vi "Config Dialog.vi"(10 "Container State":T1 caption="container state", 11 "state in":T2={"Draw Options"={"Outer Border Color"=0, "Inner Border Color"=6316128, "Outer Gradient Color"=2565927, "Inner Gradient Color"=16860, "Compass North Pointer Color"=16711680, "Compass Pointer Color 1"=13355429, "Compass Pointer Color 2"=14934973, "Direction Pointer Color"=16765184, "Text Box Outline Color"=13355429, "Text Box Background Color"=14934973, "Scale Color"=16448250, "Text Color"=0, "Draw Gradient"=TRUE, "Draw Rose"=TRUE, "Simple Scale"=TRUE, "Draw Text"=FALSE, "Font Name"="Helvetica", "Angle Units"=enum."Degrees"}} caption="State") -> (0 "state changed?":bool, 1 "data changed?":bool, 3 "state out":T2={"Draw Options"={"Outer Border Color"=0, "Inner Border Color"=6316128, "Outer Gradient Color"=2565927, "Inner Gradient Color"=16860, "Compass North Pointer Color"=16711680, "Compass Pointer Color 1"=13355429, "Compass Pointer Color 2"=14934973, "Direction Pointer Color"=16765184, "Text Box Outline Color"=13355429, "Text Box Background Color"=14934973, "Scale Color"=16448250, "Text Color"=0, "Draw Gradient"=TRUE, "Draw Rose"=TRUE, "Simple Scale"=TRUE, "Draw Text"=FALSE, "Font Name"="Helvetica", "Angle Units"=enum."Degrees"}} caption="State")   [LabVIEW 2017, in "Compass Indicator.xctl"]
uses:
  <vilib>/robotics/Controls/Compass Indicator/Compass Indicator.xctl
  <vilib>/robotics/Controls/Utilities/Color Box.ctl
  <vilib>/robotics/Controls/Compass Indicator/_Compass Indicator Support Files/Compass State.ctl
  <vilib>/robotics/Controls/Compass Indicator/Compass Picture/Draw Options.ctl
  <vilib>/robotics/Controls/Utilities/Angle Units.ctl
  <vilib>/_xctls/Container State.ctl
  <vilib>/robotics/Controls/Compass Indicator/Compass Picture/NI_Robotics_Compass Picture.lvlib
  <vilib>/_xctls/XControlSupport.lvlib
  <vilib>/robotics/Controls/Utilities/NI_Robotics_Control Utilities.lvlib
panel:
  in  "help":bool
  in  "cancel":bool
  in  "ok":bool
  in  "Angle Units":enum16{"Radians", "Degrees"}(ring)=enum."Degrees"
  out "2D Picture":picture
  in  "draw text":bool caption="Draw Text"
  in  "draw simple scale":bool=TRUE caption="Draw Simple Scale"
  in  "draw rose":bool=TRUE caption="Draw Rose"
  in  "draw grad":bool=TRUE caption="Draw Gradient"
  in  "text color":T5 caption="Text"
  in  "scale color":T5=16448250 caption="Scale"
  in  "text box bkgnd color":T5=14934973 caption="Text Box Background"
  in  "text box outline color":T5=13355429 caption="Text Box Outline"
  in  "dir ptr color":T5=16765184 caption="Direction Pointer"
  in  "compass ptr 2 color":T5=14934973 caption="Compass Pointer 2"
  in  "compass ptr1 color":T5=13355429 caption="Compass Pointer 1"
  in  "compass north ptr color":T5=16711680 caption="Compass North Pointer"
  in  "inner grad color":T5=16860 caption="Inner Gradient"
  in  "outer grad color":T5=2565927 caption="Outer Gradient"
  in  "inner border color":T5=6316128 caption="Inner Border"
  in  "outer border color":T5 caption="Outer Border"
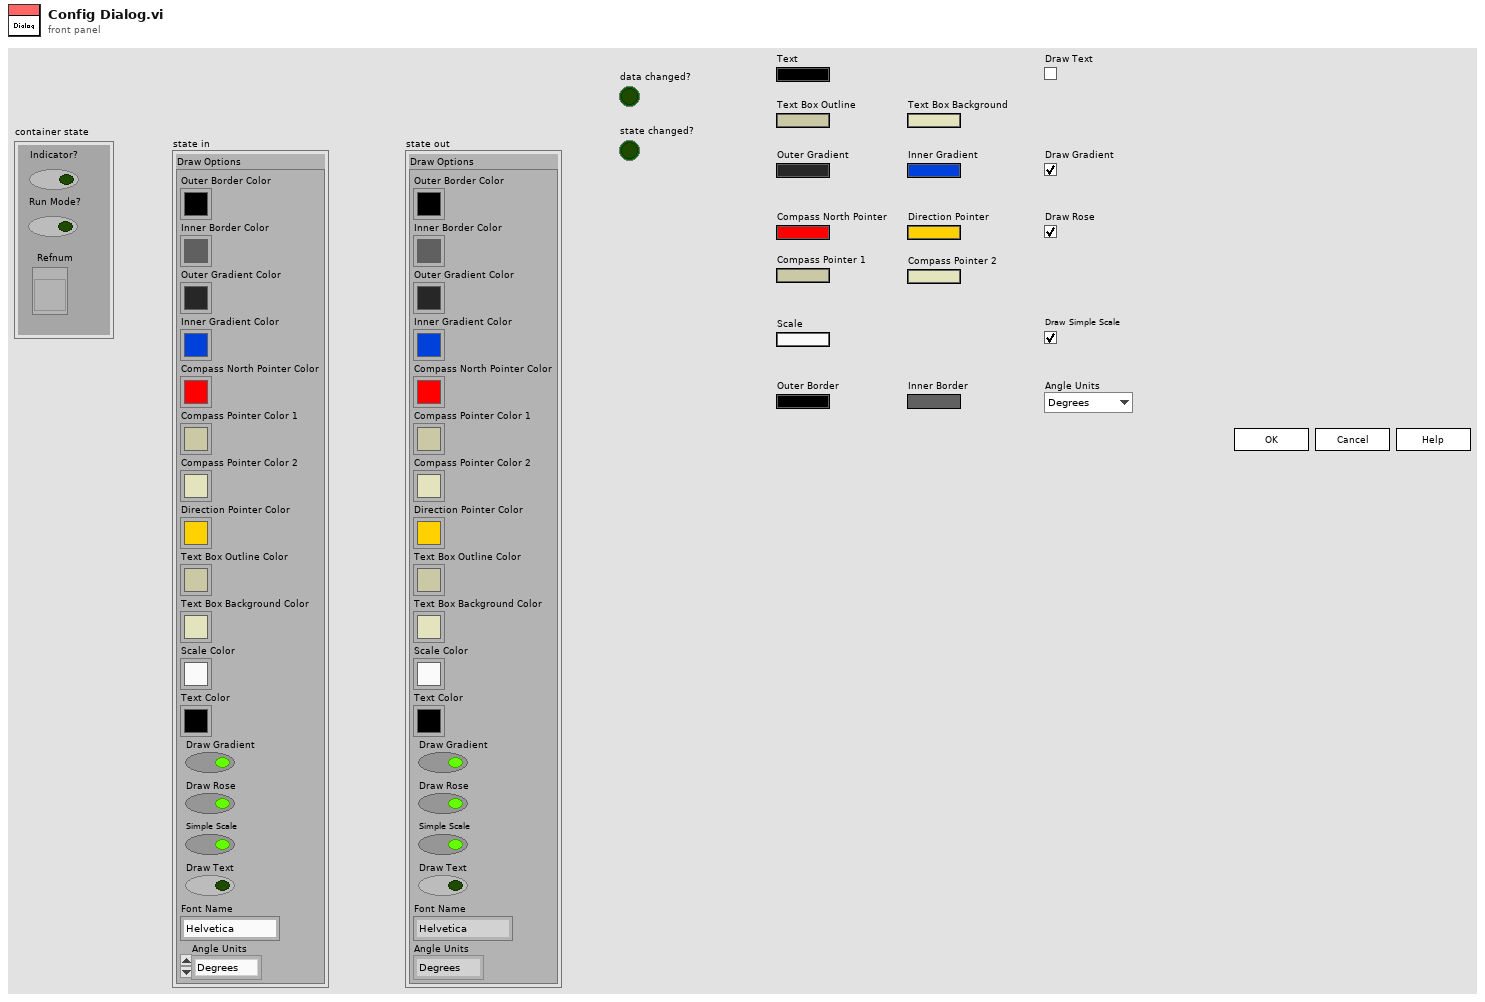
[diagram p1: front panel]
types:
  T1 = typedef "XControlSupport.lvlib/Container State.ctl" = cluster{"Indicator?":bool, "Run Mode?":bool, " Refnum":refnum<vi>}
  T2 = typedef "Compass Indicator.xctl/Compass State.ctl" = cluster{"Draw Options":T3}
  T3 = typedef "NI_Robotics_Compass Picture.lvlib/Draw Options.ctl" = cluster{"Outer Border Color":u32, "Inner Border Color":u32, "Outer Gradient Color":u32, "Inner Gradient Color":u32, "Compass North Pointer Color":u32, "Compass Pointer Color 1":u32, "Compass Pointer Color 2":u32, "Direction Pointer Color":u32, "Text Box Outline Color":u32, "Text Box Background Color":u32, "Scale Color":u32, "Text Color":u32, "Draw Gradient":bool, "Draw Rose":bool, "Simple Scale":bool, "Draw Text":bool, "Font Name":string, "Angle Units":T4}
  T4 = typedef "NI_Robotics_Control Utilities.lvlib/Angle Units.ctl" = enum16{"Radians", "Degrees"}
  T5 = typedef "NI_Robotics_Control Utilities.lvlib/Color Box.ctl" = u32
  T6 = typedef "LVBoundsTypeDef.ctl" = cluster{"Width":u32, "Height":u32}
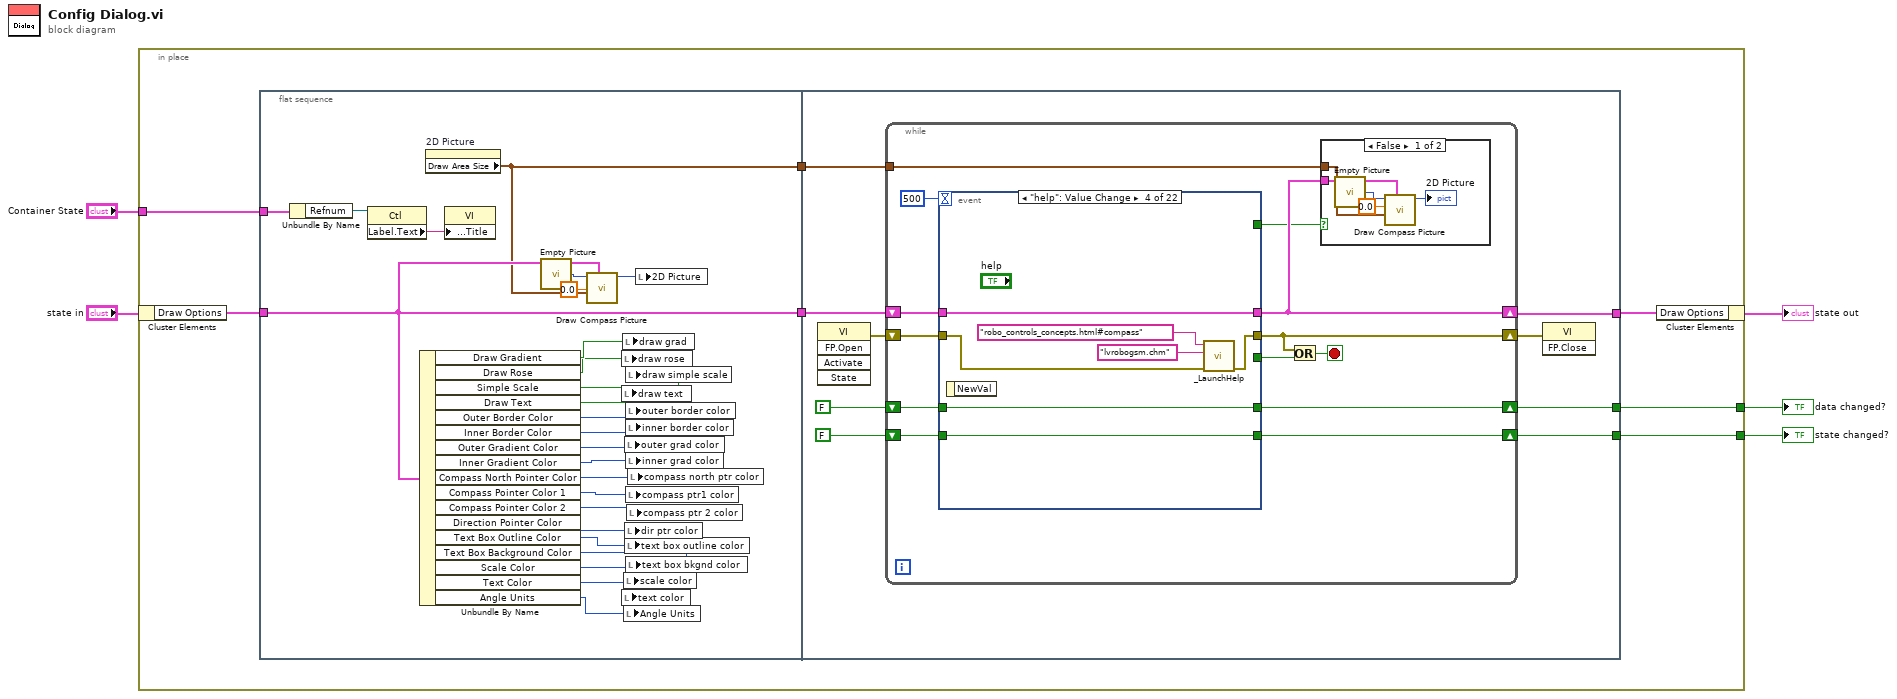
[diagram p0: block diagram]
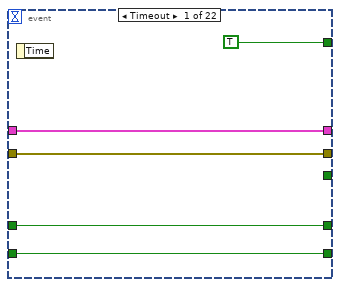
[diagram p3: hidden frame]
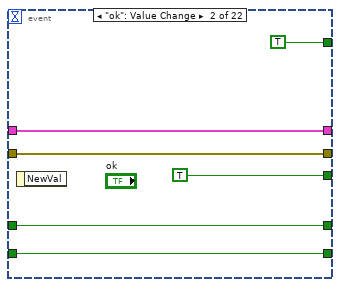
[diagram p4: hidden frame]
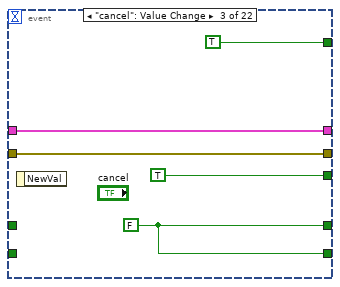
[diagram p5: hidden frame]
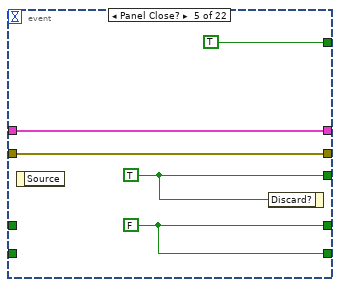
[diagram p6: hidden frame]
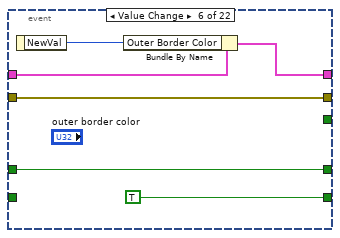
[diagram p7: hidden frame]
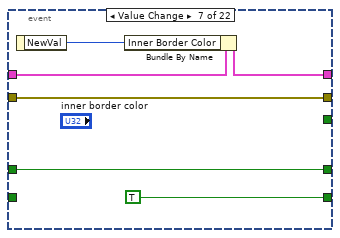
[diagram p8: hidden frame]
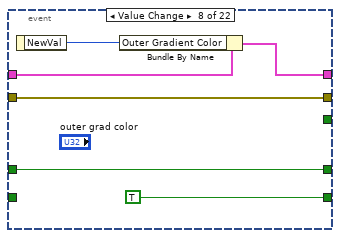
[diagram p9: hidden frame]
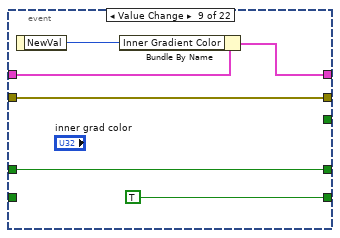
[diagram p10: hidden frame]
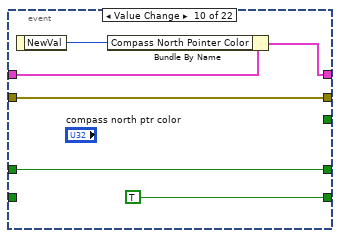
[diagram p11: hidden frame]
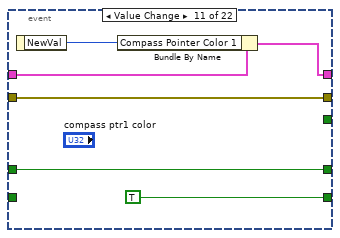
[diagram p12: hidden frame]
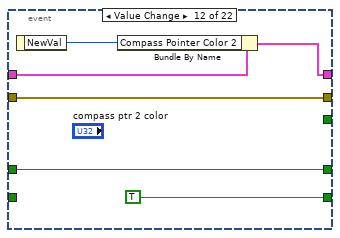
[diagram p13: hidden frame]
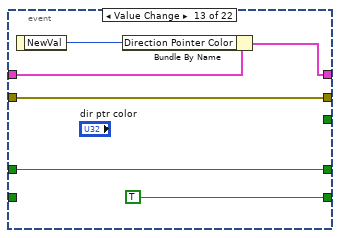
[diagram p14: hidden frame]
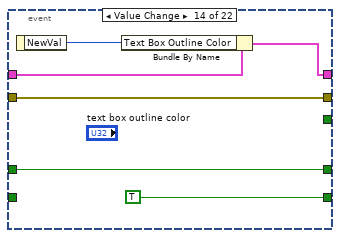
[diagram p15: hidden frame]
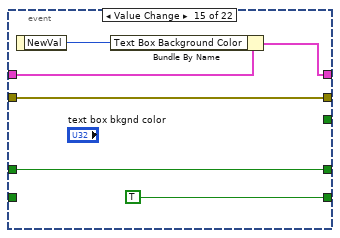
[diagram p16: hidden frame]
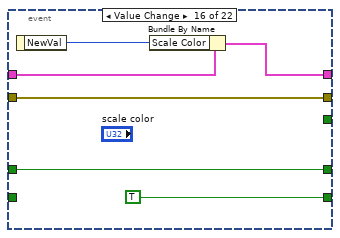
[diagram p17: hidden frame]
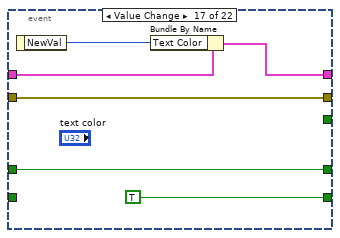
[diagram p18: hidden frame]
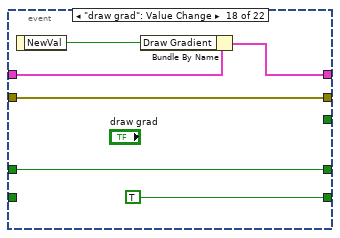
[diagram p19: hidden frame]
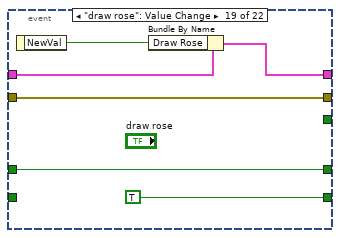
[diagram p20: hidden frame]
diagram:
  n1 = in-place {
    in-place-border: [w10] -> w5
    in-place-border: [w9] -> w4
    in-place-border: "Container State" -> [w6]
    n2 = in-place-cluster #1("state in") -> ("Draw Options"=w8:T3)
    n3 = flat-sequence {
      tunnel: w8 -> [w20]
      tunnel: [w20] -> w12
      tunnel: [w19] -> w11
      tunnel: w6 -> [w17]
      tunnel: w12 -> [w46]
      tunnel: [w43] -> w7
      tunnel: [w40] -> w10
      tunnel: [w39] -> w9
      tunnel: w11 -> [w38]
      frame #0 {
        n4 = Unbundle By Name(w17) -> ("Refnum"=w16:refnum<vi>)
        n5 = property class="Ctl"(reference=w16) -> ("Label.Text"=w15:string)  [unwired: 1 in, 2 out]
        n6 = Unbundle By Name(w20) -> ("Draw Gradient"=w37:bool, "Draw Rose"=w36:bool, "Simple Scale"=w35:bool, "Draw Text"=w34:bool, "Outer Border Color"=w33:u32, "Inner Border Color"=w32:u32, "Outer Gradient Color"=w31:u32, "Inner Gradient Color"=w30:u32, "Compass North Pointer Color"=w29:u32, "Compass Pointer Color 1"=w28:u32, "Compass Pointer Color 2"=w27:u32, "Direction Pointer Color"=w26:u32, "Text Box Outline Color"=w25:u32, "Text Box Background Color"=w24:u32, "Scale Color"=w23:u32, "Text Color"=w22:u32, "Angle Units"=w13:T4)
        n7 = property on="2D Picture" class="Pict"() -> ("Draw Area Size"=w19:T6)  [unwired: 2 in, 2 out]
        n8 = property class="VI"("Front Panel.Title"=w15) -> ()  [unwired: 2 in, 2 out]
        n9 = call "Empty Picture"() -> ("empty picture"=w18:picture)
        n10 = call <vilib>:"Draw Compass Picture.vi"("draw options"=w20, "DrawAreaSize"=w19, "angle"=0.0, "picture in"=w18) -> ("picture out"=w21:picture)  [unwired: 6 in, 1 out]
        n11 = local write "draw rose"(w36) -> ()
        n12 = local write "draw text"(w34) -> ()
        n13 = local write "text color"(w22) -> ()
        n14 = local write "draw grad"(w37) -> ()
        n15 = local write "scale color"(w23) -> ()
        n16 = local write "Angle Units"(w13) -> ()
        n17 = local write "outer grad color"(w31) -> ()
        n18 = local write "dir ptr color"(w26) -> ()
        n19 = local write "text box outline color"(w25) -> ()
        n20 = local write "draw simple scale"(w35) -> ()
        n21 = local write "outer border color"(w33) -> ()
        n22 = local write "inner border color"(w32) -> ()
        n23 = local write "inner grad color"(w30) -> ()
        n24 = local write "compass ptr1 color"(w28) -> ()
        n25 = local write "text box bkgnd color"(w24) -> ()
        n26 = local write "compass ptr 2 color"(w27) -> ()
        n27 = local write "compass north ptr color"(w29) -> ()
        n28 = local write "2D Picture"(w21) -> ()
      }
      frame #1 {
        n29 = invoke class="VI" method="FP.Open"() -> (error out=w45:errorcluster)  [unwired: 5 in, 4 out]
        n30 = while {
          shift-right: [w48] -> w43
          shift-left: w46 -> [w58]
          shift-right: [w56] -> w44
          shift-left: w45 -> [w57]
          shift-right: [w51] -> w40
          shift-left: FALSE -> [w53]
          shift-right: [w50] -> w39
          shift-left: FALSE -> [w52]
          tunnel: w38 -> [w49]
          stop <- w55 stop-if-true
          n31 = event shown="[3] \"help\": Value Change" {
            selector: _ -> [_ _ _ _ _ _ _ _ _ _ _ _ _ _ _ _ _ _ _ _ _ _]
            dyn-events: _ -> [_ _ _ _ _ _ _ _ _ _ _ _ _ _ _ _ _ _ _ _ _ _]
            timeout: 500 -> [_ _ _ _ _ _ _ _ _ _ _ _ _ _ _ _ _ _ _ _ _ _]
            tunnel: w58 -> [w69 w75 w80 w87 w92 w96 w102 w108 w114 w120 w126 w132 w138 w144 w150 w156 w162 w168 w174 w180 w186 w192]
            tunnel: w57 -> [w68 w74 w79 w82 w91 w98 w104 w110 w116 w122 w128 w134 w140 w146 w152 w158 w164 w170 w176 w182 w188 w194]
            tunnel: [w69 w75 w80 w87 w92 w95 w101 w107 w113 w119 w125 w131 w137 w143 w149 w155 w161 w167 w173 w179 w185 w191] -> w48
            tunnel: [w68 w74 w79 w81 w91 w98 w104 w110 w116 w122 w128 w134 w140 w146 w152 w158 w164 w170 w176 w182 w188 w194] -> w56
            tunnel: [_ TRUE TRUE _ w89 _ _ _ _ _ _ _ _ _ _ _ _ _ _ _ _ _] -> w54
            tunnel: w53 -> [w67 w72 _ w86 _ w97 w103 w109 w115 w121 w127 w133 w139 w145 w151 w157 w163 w169 w175 w181 w187 w193]
            tunnel: w52 -> [w66 w71 _ w85 _ _ _ _ _ _ _ _ _ _ _ _ _ _ _ _ _ _]
            tunnel: [w67 w72 w78 w86 w90 w97 w103 w109 w115 w121 w127 w133 w139 w145 w151 w157 w163 w169 w175 w181 w187 w193] -> w51
            tunnel: [w66 w71 w78 w85 w90 TRUE TRUE TRUE TRUE TRUE TRUE TRUE TRUE TRUE TRUE TRUE TRUE TRUE TRUE TRUE TRUE TRUE] -> w50
            tunnel: [TRUE TRUE TRUE _ TRUE _ _ _ _ _ _ _ _ _ _ _ _ _ _ _ _ _] -> w47
            event Timeout {
              n32 = event-data() -> ()  [unwired: 1 in, 1 out]
            }
            event "ok": Value Change {
              n33 = event-data() -> ()  [unwired: 1 in, 1 out]
            }
            event "cancel": Value Change {
              w78 = FALSE
              n34 = event-data() -> ()  [unwired: 1 in, 1 out]
            }
            event "help": Value Change {
              n35 = event-data() -> ()  [unwired: 1 in, 1 out]
              n36 = call <helpdir>:"_LaunchHelp.vi"("error in (no error)"=w82, "CHM or HLP filename (lvdialog.chm)"="lvrobogsm.chm", "HTML filename"="robo_controls_concepts.html#compass") -> ("error out"=w81:errorcluster)  [unwired: 4 out]
            }
            event Panel Close? {
              w89 = TRUE
              w90 = FALSE
              n37 = event-data() -> ()  [unwired: 1 in, 1 out]
              n38 = event-data("Discard?"=w89) -> ()  [unwired: 1 in, 1 out]
            }
            event Value Change {
              n39 = event-data() -> ("NewVal"=w94:T5)  [unwired: 1 in]
              n40 = Bundle By Name(cluster=w96, "Outer Border Color"=w94) -> (w95:T3)
            }
            event Value Change {
              n41 = event-data() -> ("NewVal"=w100:T5)  [unwired: 1 in]
              n42 = Bundle By Name(cluster=w102, "Inner Border Color"=w100) -> (w101:T3)
            }
            event Value Change {
              n43 = event-data() -> ("NewVal"=w106:T5)  [unwired: 1 in]
              n44 = Bundle By Name(cluster=w108, "Outer Gradient Color"=w106) -> (w107:T3)
            }
            event Value Change {
              n45 = event-data() -> ("NewVal"=w112:T5)  [unwired: 1 in]
              n46 = Bundle By Name(cluster=w114, "Inner Gradient Color"=w112) -> (w113:T3)
            }
            event Value Change {
              n47 = event-data() -> ("NewVal"=w118:T5)  [unwired: 1 in]
              n48 = Bundle By Name(cluster=w120, "Compass North Pointer Color"=w118) -> (w119:T3)
            }
            event Value Change {
              n49 = event-data() -> ("NewVal"=w124:T5)  [unwired: 1 in]
              n50 = Bundle By Name(cluster=w126, "Compass Pointer Color 1"=w124) -> (w125:T3)
            }
            event Value Change {
              n51 = event-data() -> ("NewVal"=w130:T5)  [unwired: 1 in]
              n52 = Bundle By Name(cluster=w132, "Compass Pointer Color 2"=w130) -> (w131:T3)
            }
            event Value Change {
              n53 = event-data() -> ("NewVal"=w136:T5)  [unwired: 1 in]
              n54 = Bundle By Name(cluster=w138, "Direction Pointer Color"=w136) -> (w137:T3)
            }
            event Value Change {
              n55 = event-data() -> ("NewVal"=w142:T5)  [unwired: 1 in]
              n56 = Bundle By Name(cluster=w144, "Text Box Outline Color"=w142) -> (w143:T3)
            }
            event Value Change {
              n57 = event-data() -> ("NewVal"=w148:T5)  [unwired: 1 in]
              n58 = Bundle By Name(cluster=w150, "Text Box Background Color"=w148) -> (w149:T3)
            }
            event Value Change {
              n59 = event-data() -> ("NewVal"=w154:T5)  [unwired: 1 in]
              n60 = Bundle By Name(cluster=w156, "Scale Color"=w154) -> (w155:T3)
            }
            event Value Change {
              n61 = event-data() -> ("NewVal"=w160:T5)  [unwired: 1 in]
              n62 = Bundle By Name(cluster=w162, "Text Color"=w160) -> (w161:T3)
            }
            event "draw grad": Value Change {
              n63 = event-data() -> ("NewVal"=w166:bool)  [unwired: 1 in]
              n64 = Bundle By Name(cluster=w168, "Draw Gradient"=w166) -> (w167:T3)
            }
            event "draw rose": Value Change {
              n65 = event-data() -> ("NewVal"=w172:bool)  [unwired: 1 in]
              n66 = Bundle By Name(cluster=w174, "Draw Rose"=w172) -> (w173:T3)
            }
            event "draw simple scale": Value Change {
              n67 = event-data() -> ("NewVal"=w178:bool)  [unwired: 1 in]
              n68 = Bundle By Name(cluster=w180, "Simple Scale"=w178) -> (w179:T3)
            }
            event "draw text": Value Change {
              n69 = event-data() -> ("NewVal"=w184:bool)  [unwired: 1 in]
              n70 = Bundle By Name(cluster=w186, "Draw Text"=w184) -> (w185:T3)
            }
            event "Angle Units": Value Change {
              n71 = event-data() -> ("NewVal"=w190:enum16{"Radians", "Degrees"})  [unwired: 1 in]
              n72 = Bundle By Name(cluster=w192, "Angle Units"=w190) -> (w191:T3)
            }
          }
          n73 = Or(x=w56, y=w54) -> (x .or. y?=w55:bool)
          n74 = case shown="False" w47 {
            tunnel: w49 -> [w62 _]
            tunnel: w48 -> [w63 _]
            frame False {
              n75 = call "Empty Picture"() -> ("empty picture"=w61:picture)
              n76 = call <vilib>:"Draw Compass Picture.vi"("draw options"=w63, "DrawAreaSize"=w62, "angle"=0.0, "picture in"=w61) -> ("picture out"=→"2D Picture":picture)  [unwired: 6 in, 1 out]
            }
            frame True {
            }
          }
        }
        n77 = invoke class="VI" method="FP.Close"(error in=w44) -> ()  [unwired: 2 in, 3 out]
      }
    }
    n78 = in-place-cluster #1("Draw Options"=w7) -> (→"state out":T2)
  }
  "data changed?" <- w5
  "state changed?" <- w4
